vi "default document.vi"() -> (4 "Device Out":T1, 6 "Comm":T2, 15 "error out":errorcluster)   [LabVIEW 2019]
uses:
  <userlib>/IoT Devices/_subVIs/HTTPComm.ctl
  <userlib>/Onshape/_SubVI/Cluster.ctl
panel:
  in  "Device In":T1
  in  "error in":errorcluster
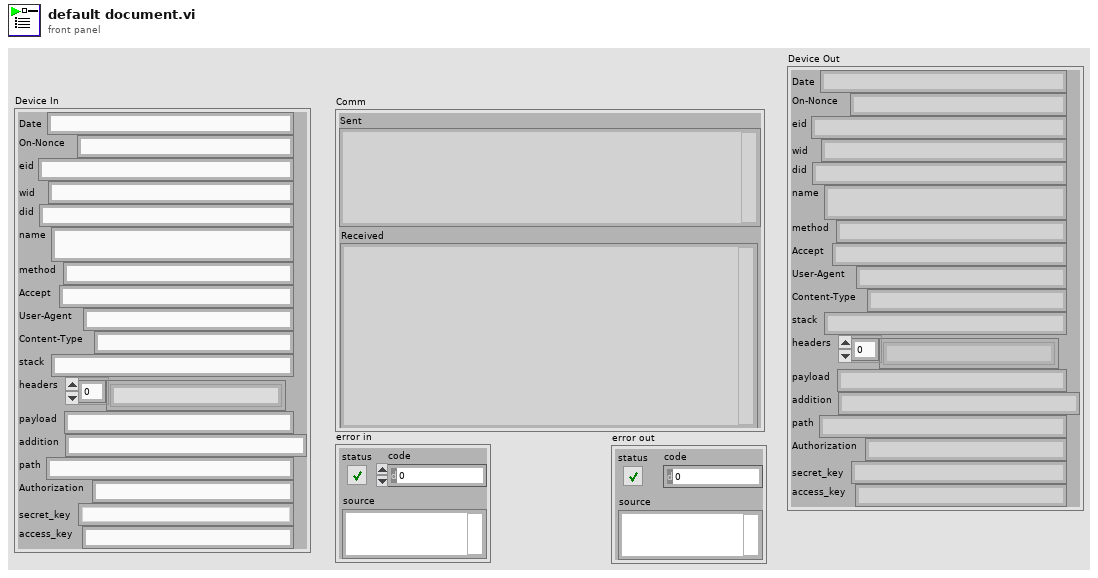
[diagram p1: front panel]
types:
  T1 = typedef "Cluster.ctl" = cluster{"Date":string, "On-Nonce":string, "eid":string, "wid":string, "did":string, "name":string, "method":string, "Accept":string, "User-Agent":string, "Content-Type":string, "stack":string, "headers":string[], "payload":string, "addition":string, "path":string, "Authorization":string, "secret_key":string, "access_key":string}
  T2 = typedef "HTTPComm.ctl" = cluster{"url":string, "sent headers":string, "sent body":string, "headers":string, "body":string, "Sent":string, "Received":string}
  T3 = cluster{"items":cluster{"resourceType":string, "id":string, "name":string, "defaultWorkspace":cluster{"id":string}}[]}
  T4 = cluster{"resourceType":string, "id":string, "name":string, "defaultWorkspace":cluster{"id":string}}[]
  T5 = cluster{"resourceType":string, "id":string, "name":string, "defaultWorkspace":cluster{"id":string}}
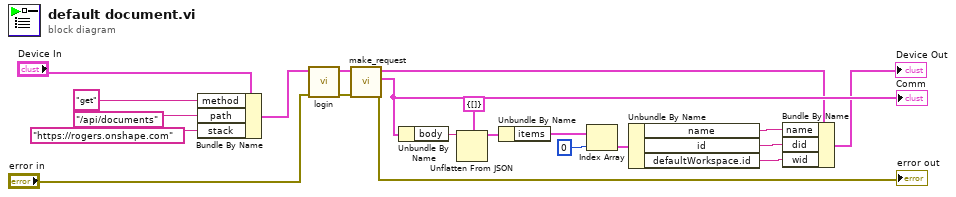
[diagram p0: block diagram]
diagram:
  n1 = Bundle By Name(cluster="Device In", "method"="get" ("Method"), "path"="/api/documents" ("payload"), "stack"="https://rogers.onshape.com" ("stacks")) -> (w2:T1)
  n2 = call <userlib>:"login.vi"("error in"="error in", "Device In"=w2) -> ("error out"=w12:errorcluster, "Device Out"=w11:T1)  [unwired: 8 in]
  n3 = call <userlib>:"make_request.vi"("Error in"=w12, "Device In"=w11) -> ("error out"=→"error out":errorcluster, "Comm"=w17:T2, "Device Out"=w7:T1)  [unwired: 5 in, 2 out]
  "Comm" <- w17
  n4 = Unbundle By Name(w17) -> ("body"=w16:string)
  n5 = Unflatten From JSON(JSON string=w16, type and defaults=T3 {"items"=[]}) -> (value=w14:T3)  [unwired: 5 in, 1 out]
  n6 = Unbundle By Name(w14) -> ("items"=w10:T4)
  n7 = Index Array(array=w10, index=0) -> (element=w8:T5)
  n8 = Unbundle By Name(w8) -> ("name"=w6:string, "id"=w5:string, "defaultWorkspace.id"=w4:string)
  n9 = Bundle By Name(cluster=w7, "name"=w6, "did"=w5, "wid"=w4) -> (→"Device Out":T1)
